vi "XY Galvo With Homography.v3.vi"(1 "Microscope Settings in":T2={"Mode"=enum."X", "Slit"={"Scanning Mode"=0.0, "Slit Width /%"=0.0}, "Colour Channel"=enum."3", "Colour"=[], "Exposure/ms"=0.0, "Piezo Position /um"=0.0, "ROI"={"X"={"Start /px"=0.0, "Step /px"=0.0, "Range /px"=0.0}, "Y"={"Start /px"=0.0, "Step /px"=0.0, "Range /px"=0.0}, "Z "={"Start /um"=0.0, "Step/um"=0.0, "Range /um"=0.0}, "T "={"Start /s"=0.0, "Step /s"=1.0, "Range /s"=100.0}}, "Samples per millisecond"=0.0, "Relax/ms"=0.0, "Readout Direction"=0.0, "Trigger Source"=0.0, "Camera Delay /ms"=0.0, "Under Scan /ms"=0.0, "Slit Delay"=100.0, "Waveforms"={"Analogue Out"=[{"t0"=timestamp(0 s since 1904-01-01), "dt"=1.0, "Y"=[]}, {"t0"=timestamp(0 s since 1904-01-01), "dt"=1.0, "Y"=[]}, {"t0"=timestamp(0 s since 1904-01-01), "dt"=1.0, "Y"=[]}], "Digital Out"=[{"t0"=timestamp(0 s since 1904-01-01), "dt"=0.0, "Y"={"transitions"=[], "data"=[]}}, {"t0"=timestamp(0 s since 1904-01-01), "dt"=0.0, "Y"={"transitions"=[], "data"=[]}}, {"t0"=timestamp(0 s since 1904-01-01), "dt"=0.0, "Y"={"transitions"=[], "data"=[]}}]}} {"Under Scan /ms" min=0.0 max=10.0 step=0.05; "ROI"."T"."Range /s" min=0.0 max=10.0 step=0.05; "ROI"."T"."Step /s" min=0.0 max=10.0 step=0.05; "ROI"."T"."Start /s" min=0.0 max=10.0 step=0.05; "ROI"."X"."Range /px" min=0.0 max=10.0 step=0.05; "ROI"."X"."Step /px" min=0.0 max=10.0 step=0.05; "ROI"."X"."Start /px" min=0.0 max=10.0 step=0.05; "ROI"."Y"."Range /px" min=0.0 max=10.0 step=0.05; "ROI"."Y"."Step /px" min=0.0 max=10.0 step=0.05; "ROI"."Y"."Start /px" min=0.0 max=10.0 step=0.05; "ROI"."Z"."Range /um" min=0.0 max=10.0 step=0.05; "ROI"."Z"."Step/um" min=0.0 max=10.0 step=0.05; "ROI"."Z"."Start /um" min=0.0 max=10.0 step=0.05; "Colour"."Focus Offset /um" min=0.0 max=10.0 step=0.05 scale=-100.0..20.0 scale format="%.2f"; "Colour"."Colour"."Filter" items=["Empty"=1, ""=2, ""=3, "561"=4, ""=5, "488"=6]; "Camera Delay /ms" min=0.0 max=10.0 step=0.05; "Trigger Source" items=["Internal"=1.0, "External"=2.0]; "Readout Direction" items=["Forward"=1.0, "Backward"=2.0]; "Slit"."Scanning Mode" items=["Full Frame"=1.0, "Slit Scanning"=12.0]; "Piezo Position /um" min=0.0 max=10.0 step=0.05; "Exposure/ms" min=0.0 max=10.0 step=0.05; "Relax/ms" min=1.0 max=2.0 step=1.0}, 2 "Colour Channel":dbl) -> (0 "Signals":T1(graph))   [LabVIEW 2016]
uses:
  controls/Microscope Settings.ctl
  controls/ColourCalibration.ctl
  <vilib>/Analysis/NI_AALBase.lvlib
panel:
  out "Underscan /ms":dbl
  out "Prexposure /ms":dbl
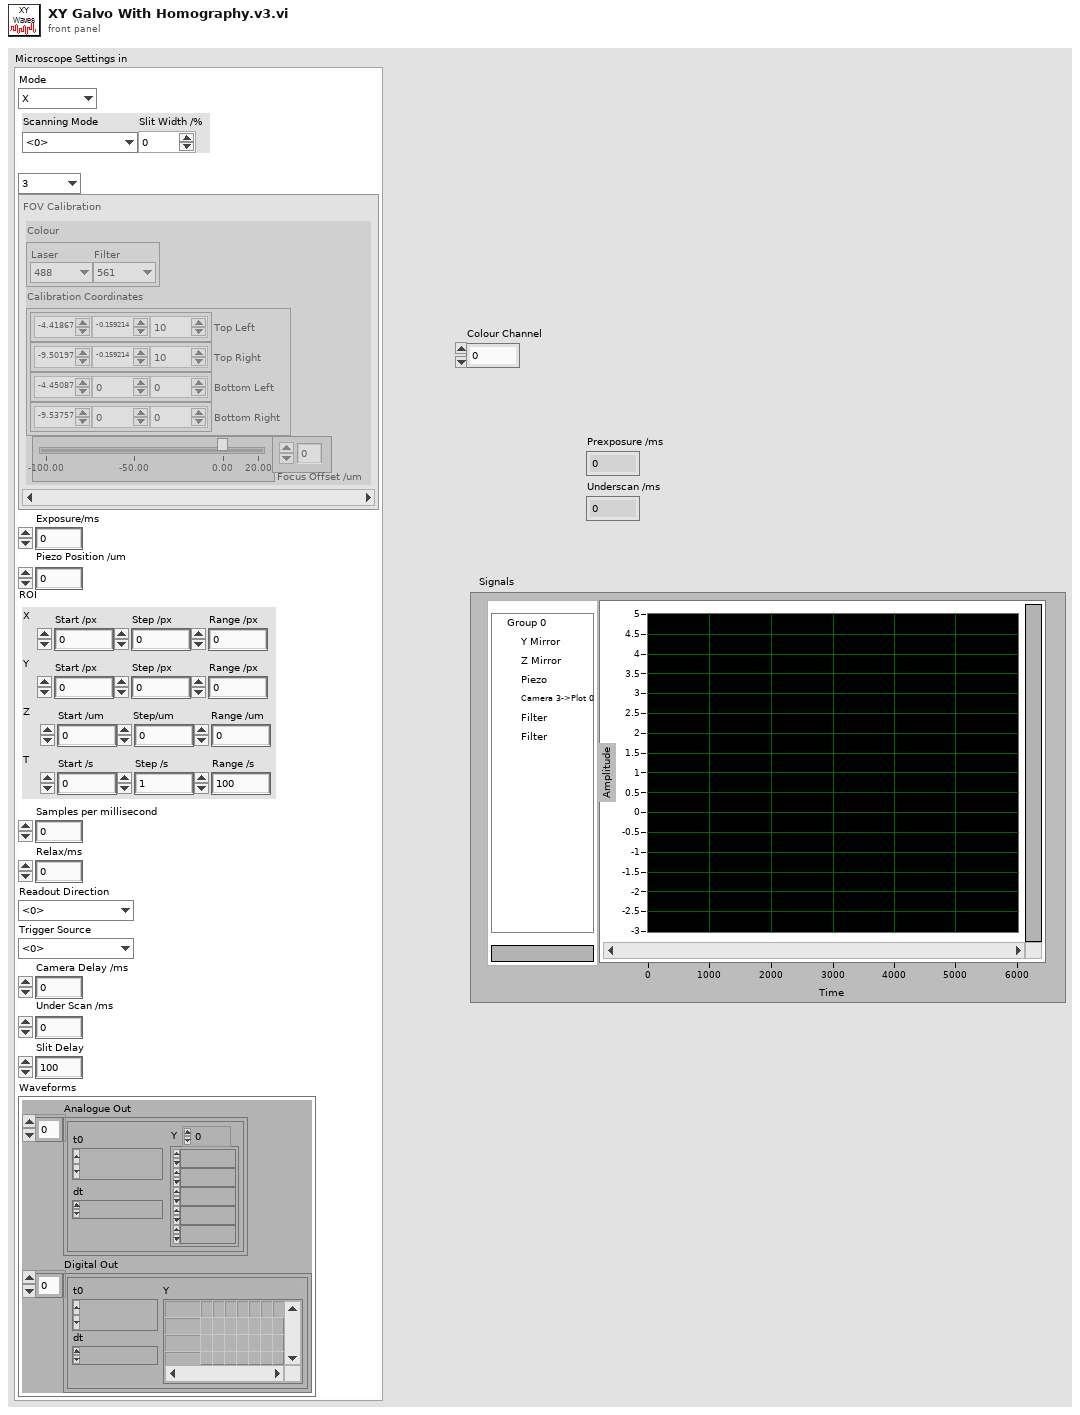
[diagram p1: front panel]
types:
  T1 = cluster{"Y Mirror":dbl[], "Z Mirror":dbl[], "Piezo":dbl[], "Camera":dbl[], "Laser":dbl[], "Laser 2":dbl[]}
  T2 = typedef "Microscope Settings.ctl" = cluster{"Mode":enum16{"Brightfield", "X", "XY", "XYZ", "XYC", "XYCT", "XYZT", "XYZC", "Tweezers", "Virus"}, "Slit":cluster{"Scanning Mode":dbl, "Slit Width /%":dbl}, "Colour Channel":enum16{"1", "2", "3", "4", "5"}, "Colour":T3, "Exposure/ms":dbl, "Piezo Position /um":dbl, "ROI":cluster{"X":cluster{"Start /px":dbl, "Step /px":dbl, "Range /px":dbl}, "Y":cluster{"Start /px":dbl, "Step /px":dbl, "Range /px":dbl}, "Z ":cluster{"Start /um":dbl, "Step/um":dbl, "Range /um":dbl}, "T ":cluster{"Start /s":dbl, "Step /s":dbl, "Range /s":dbl}}, "Samples per millisecond":dbl, "Relax/ms":dbl, "Readout Direction":dbl, "Trigger Source":dbl, "Camera Delay /ms":dbl, "Under Scan /ms":dbl, "Slit Delay":dbl, "Waveforms":cluster{"Analogue Out":waveform(dbl)[], "Digital Out":digitalwaveform[]}}
  T3 = typedef "ColourCalibration.ctl" = cluster{"Colour":cluster{"Laser":enum16{"Brightfield", "445", "488", "561", "647"}, "Filter":u16}, "Calibration Coordinates":cluster{"Top Left":dbl[], "Top Right":dbl[], "Bottom Left":dbl[], "Bottom Right":dbl[]}, "Focus Offset /um":dbl}[]
  T4 = cluster{"Y Mirror":dbl[], "Z Mirror":dbl[], "Piezo":dbl[], "Camera":dbl[], "Laser":dbl[], "Filter":dbl[]}
  T5 = cluster{"X":cluster{"Start /px":dbl, "Step /px":dbl, "Range /px":dbl}, "Y":cluster{"Start /px":dbl, "Step /px":dbl, "Range /px":dbl}, "Z ":cluster{"Start /um":dbl, "Step/um":dbl, "Range /um":dbl}, "T ":cluster{"Start /s":dbl, "Step /s":dbl, "Range /s":dbl}}
  T6 = cluster{"Start /px":dbl, "Step /px":dbl, "Range /px":dbl}
  T7 = cluster{"Colour":cluster{"Laser":enum16{"Brightfield", "445", "488", "561", "647"}, "Filter":u16}, "Calibration Coordinates":cluster{"Top Left":dbl[], "Top Right":dbl[], "Bottom Left":dbl[], "Bottom Right":dbl[]}, "Focus Offset /um":dbl}
  T8 = cluster{"Top Left":dbl[], "Top Right":dbl[], "Bottom Left":dbl[], "Bottom Right":dbl[]}
  T9 = typedef "NI_Matrix.lvlib/RealMatrix.ctl" = dbl[][]
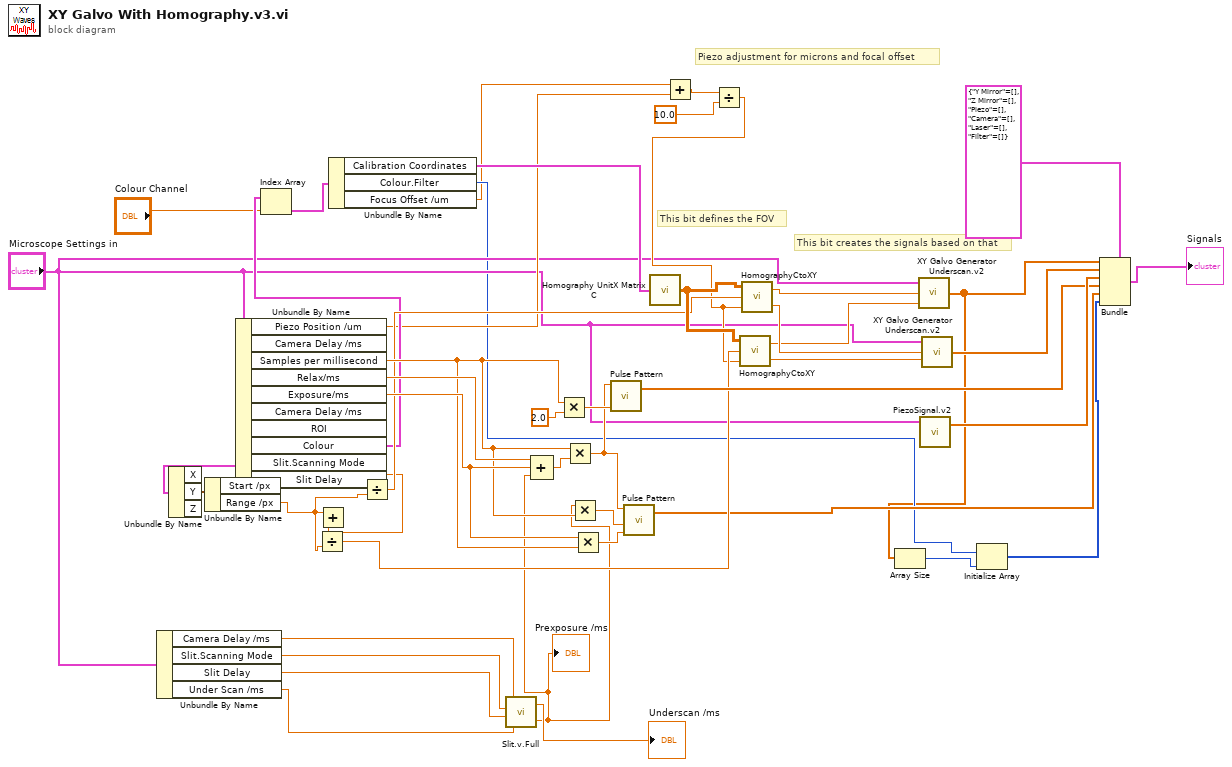
[diagram p0: block diagram]
diagram:
  # "Piezo adjustment for microns and focal offset"
  # "This bit creates the signals based on that"
  # "This bit defines the FOV"
  n1 = Unbundle By Name("Microscope Settings in") -> ("Camera Delay /ms"=w12:dbl, "Slit.Scanning Mode"=w13:dbl, "Slit Delay"=w10:dbl, "Under Scan /ms"=w11:dbl)
  n2 = Unbundle By Name("Microscope Settings in") -> ("Piezo Position /um"=w15:dbl, "Samples per millisecond"=w36:dbl, "Relax/ms"=w43:dbl, "Exposure/ms"=w37:dbl, "ROI"=w28:T5, "Colour"=w21:T3)  [unwired: 4 out]
  n3 = Unbundle By Name(w28) -> ("Y"=w27:T6)  [unwired: 2 out]
  n4 = Unbundle By Name(w27) -> ("Start /px"=w24:dbl, "Range /px"=w22:dbl)
  n5 = Index Array(array=w21, index="Colour Channel") -> (element=w19:T7)
  n6 = Add(x=w22, y=w24) -> (x+y=w23:dbl)
  n7 = Divide(x=w23, y=w22) -> (x/y=w25:dbl)
  n8 = Unbundle By Name(w19) -> ("Calibration Coordinates"=w16:T8, "Colour.Filter"=w4:u16, "Focus Offset /um"=w1:dbl)
  n9 = Divide(x=w24, y=w22) -> (x/y=w26:dbl)
  n10 = call "Slit.v.Full.vi"("Under Scan /ms"=w11, "Slit Delay"=w10, "Scanning Mode"=w13, "Camera Delay /ms"=w12) -> ("Prexposure /ms"=w7:dbl, "Underscan /ms"=→"Underscan /ms":dbl)
  "Prexposure /ms" <- w7
  n11 = Compound Arithmetic op=ADD(w43, w37, w7) -> (w42:dbl)
  n12 = Multiply(x=w36, y=2.0) -> (x*y=w40:dbl)
  n13 = Multiply(x=w36, y=w42) -> (x*y=w39:dbl)
  n14 = Multiply(x=w7, y=w36) -> (x*y=w38:dbl)
  n15 = Multiply(x=w37, y=w36) -> (x*y=w35:dbl)
  n16 = call <vilib>:"Pulse Pattern.vi"("width"=w40, "samples"=w39) -> ("Pulse Pattern"=w41:dbl[])  [unwired: 2 in, 1 out]
  n17 = call <vilib>:"Pulse Pattern.vi"("width"=w35, "delay"=w38, "samples"=w39) -> ("Pulse Pattern"=w6:dbl[])  [unwired: 1 in, 1 out]
  n18 = call "Homography UnitX Matrix C.vi"("input cluster"=w16) -> ("C"=w45:T9)
  n19 = Add(x=w1, y=w15) -> (x+y=w14:dbl)
  n20 = Divide(x=w14, y=10.0) -> (x/y=w17:dbl)
  n21 = call "HomographyCtoXY.vi"("Y"=w17, "X"=w25, "C"=w45) -> ("Y"=w29:dbl, "X"=w30:dbl)
  n22 = call "HomographyCtoXY.vi"("Y"=w17, "X"=w26, "C"=w45) -> ("Y"=w32:dbl, "X"=w31:dbl)
  n23 = call "XY Galvo Generator Underscan.v2.vi"("FOV max / V"=w30, "FOV min/ V"=w31, "Microscope Settings in"="Microscope Settings in") -> ("XY Galvo"=w2:dbl[])
  n24 = Array Size(array=w2) -> (size(s)=w5:i32)
  n25 = call "PiezoSignal.v2.vi"("Microscope Settings in"="Microscope Settings in") -> ("Piezo Signal"=w46:dbl[])  [unwired: 3 in]
  n26 = call "XY Galvo Generator Underscan.v2.vi"("FOV max / V"=w29, "FOV min/ V"=w32, "Microscope Settings in"="Microscope Settings in") -> ("XY Galvo"=w47:dbl[])
  n27 = Initialize Array(w4, w5) -> (w3:u16[])
  n28 = Bundle(cluster=T4 {"Y Mirror"=[], "Z Mirror"=[], "Piezo"=[], "Camera"=[], "Laser"=[], "Filter"=[]}, "Y Mirror"=w2, "Z Mirror"=w47, "Piezo"=w46, "Camera"=w41, "Laser"=w6, "Filter"=w3) -> (→"Signals":T4)
